vi "PipBoy_UpdateFileConf.vi"(8 "error in (no error)":errorcluster, 10 "FileConf":T1) -> (0 "error out":errorcluster)   [LabVIEW 2014]
uses:
  ctls/PipBoy_FileConf.ctl
  <vilib>/Utility/config.llb/NI_LVConfig.lvlib
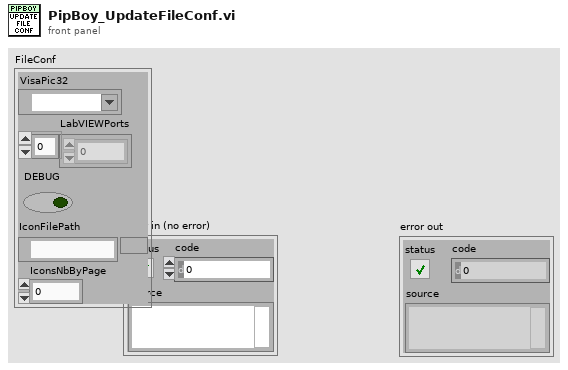
[diagram p1: front panel]
types:
  T1 = typedef "PipBoy_FileConf.ctl" = cluster{"VisaPic32":refnum<visa-resource-name>, "LabVIEWPorts":u16[], "DEBUG":bool, "IconFilePath":path, "IconsNbByPage":i32}
  T2 = typedef "NI_LVConfig.lvlib/Config Data RefNum.ctl" = refnum<k1>
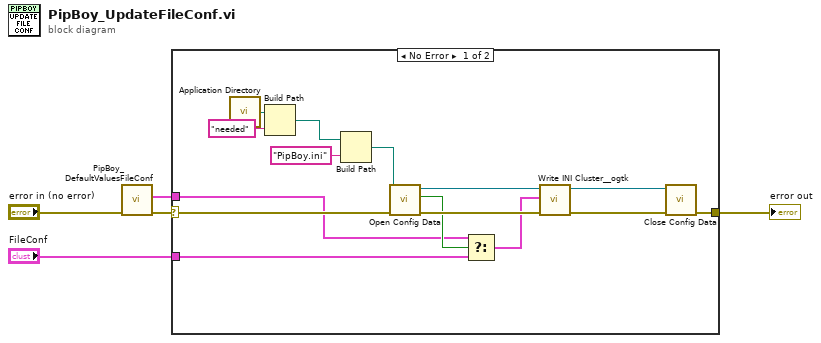
[diagram p0: block diagram]
diagram:
  n1 = call "PipBoy_DefaultValuesFileConf.vi"("error in (no error)"="error in (no error)") -> ("error out"=w2:errorcluster, "FileConf"=w4:T1)  [unwired: 9 in]
  n2 = case shown="No Error" w2 {
    selector: w2 -> [w10 w21]
    tunnel: [w14 w21] -> w5
    tunnel: w4 -> [w7 _]
    tunnel: "FileConf" -> [w8 _]
    frame No Error {
      n3 = call <vilib>:"Application Directory.vi"() -> ("Application Directory"=w20:path)
      n4 = Build Path(base path=w20, name or relative path="needed") -> (appended path=w18:path)
      n5 = Build Path(base path=w18, name or relative path="PipBoy.ini") -> (appended path=w16:path)
      n6 = call <vilib>:"Open Config Data.vi"("error in (no error)"=w10, "configuration file path"=w16) -> ("error out"=w15:errorcluster, "file created?"=w9:bool, "refnum"=w11:T2)  [unwired: 7 in]
      n7 = Select(t=w7, s=w9, f=w8) -> (s? t:f=w6:T1)
      n8 = call <userlib>:"Write INI Cluster__ogtk.vi"("error in (no error)"=w15, "INI Fomatted Cluster"=w6, "refnum"=w11) -> ("error out"=w13:errorcluster, "dup refnum"=w12:T2)  [unwired: 7 in]
      n9 = call <vilib>:"Close Config Data.vi"("error in (no error)"=w13, "refnum"=w12) -> ("error out"=w14:errorcluster)  [unwired: 8 in, 1 out]
    }
    frame Error {
    }
  }
  "error out" <- w5
